vi "AlliGator Extrapolate Multiple Plots.vi"(8 "error in (no error)":errorcluster, 10 "Selected Plots":i32[](array[numeric]), 11 "Selected Plot Info":T1) -> (0 "error out":errorcluster, 1 "Extrapolated Decay Message":string, 3 "Last Extrapolated Decay":cluster{"t Array":dbl[], "IRF Array":dbl[]}, 4 "Single Plot?":bool)   [LabVIEW 2021, in "AlliGator Decay Analysis.lvlib" / "AlliGator Decay Processing.lvlib"]
doc: "Extrapolated the selected plots."
uses:
  AlliGator Decay Processing.lvlib
  Graphs/XY Graph/XY Graph Selected Plot Info.ctl
  Graphs/XY Graph/XY Graph Refnum.ctl
  <vilib>/Utility/miscctls.llb/LVPoint32TypeDef.ctl
  Strings/Strings.lvlib
  AlliGator Decay Preprocessing.lvlib
  Graphs/XY Graph/XY Graph Add-Ons.lvlib
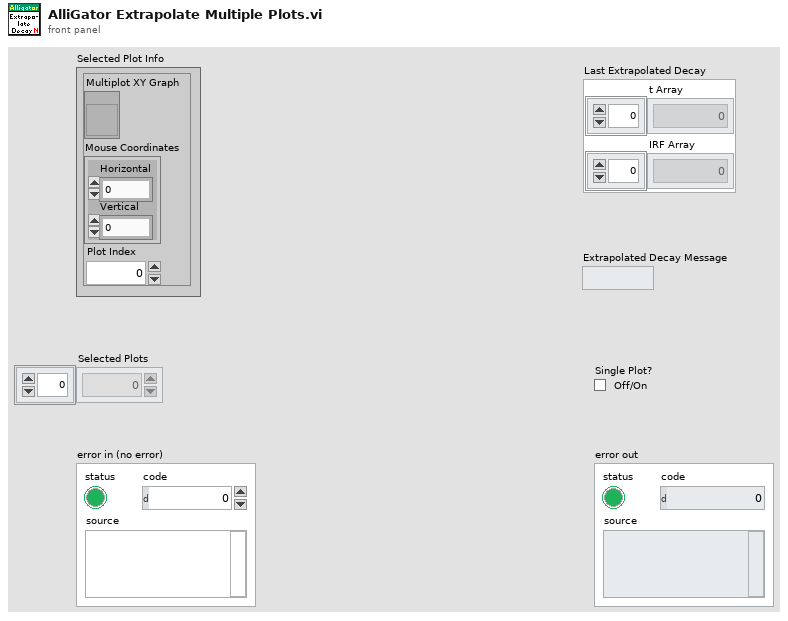
[diagram p1: front panel]
types:
  T1 = typedef "XY Graph Add-Ons.lvlib/XY Graph Selected Plot Info.ctl" = cluster{"Multiplot XY Graph":T2, "Mouse Coordinates":T3, "Plot Index":i32}
  T2 = typedef "XY Graph Add-Ons.lvlib/XY Graph Refnum.ctl" = refnum<vi>
  T3 = typedef "LVPoint32TypeDef.ctl" = cluster{"Horizontal":i32, "Vertical":i32}
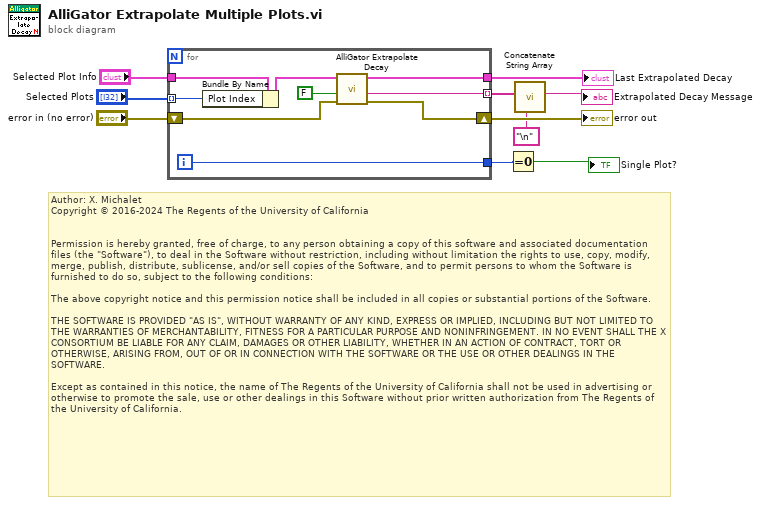
[diagram p0: block diagram]
diagram:
  # "Author: X. Michalet\nCopyright © 2016-2024 The Regents of the University of California\n \n\nPermission is hereby granted, free of charge, to any person obtaining a copy of this software and associated documentation files (the \"Software\"), to deal in the Software without restriction, including without limitation the rights to use, copy, modify, merge, publish, distribute, sublicense, and/or sell copies of the Software, and to permit persons to whom the Software is furnished to do so, subject to the following conditions:\n\nThe above copyright notice and this permission notice shall be included in all copies or substantial portions of the Software.\n\nTHE SOFTWARE IS PROVIDED \"AS IS\", WITHOUT WARRANTY OF ANY KIND, EXPRESS OR IMPLIED, INCLUDING BUT NOT LIMITED TO THE WARRANTIES OF MERCHANTABILITY, FITNESS FOR A PARTICULAR PURPOSE AND NONINFRINGEMENT. IN NO EVENT SHALL THE X CONSORTIUM BE LIABLE FOR ANY CLAIM, DAMAGES OR OTHER LIABILITY, WHETHER IN AN ACTION OF CONTRACT, TORT OR OTHERWISE, ARISING FROM, OUT OF OR IN CONNECTION WITH THE SOFTWARE OR THE USE OR OTHER DEALINGS IN THE SOFTWARE.\n\nExcept as contained in this notice, the name of The Regents of the University of California shall not be used in advertising or otherwise to promote the sale, use or other dealings in this Software without prior written authorization from The Regents of the University of California."
  n1 = for {
    tunnel: "Selected Plot Info" -> [w19]
    tunnel: [w17] -> w5 mode=indexing
    tunnel: [w15] -> w7
    shift-right: [w16] -> w8
    shift-left: "error in (no error)" -> [w18]
    tunnel: "Selected Plots" -> [w13] mode=indexing
    tunnel: [w12] -> w2
    i -> [w12]
    n2 = Bundle By Name(cluster=w19, "Plot Index"=w13) -> (w14:T1)
    n3 = call "AlliGator Extrapolate Decay.vi"("error in (no error)"=w18, "Replace Plot (T)?"=FALSE, "Selected Plot Info"=w14) -> ("Error Out"=w16:errorcluster, "Message"=w17:string, "Extrapolated Decay"=w15:cluster{"t Array":dbl[], "IRF Array":dbl[]})  [unwired: 6 in]
  }
  "error out" <- w8
  "Last Extrapolated Decay" <- w7
  n4 = Equal To 0?(x=w2) -> (x = 0?=→"Single Plot?":bool)
  n5 = call "Concatenate String Array.vi"("Separator (TAB)"="\n", "String Array"=w5) -> ("Formatted String"=→"Extrapolated Decay Message":string)  [unwired: 9 in]
